vi "Add Default Enum.vi"(6 "Hdr Name":T1, 8 "error in (no error)":errorcluster, 9 "Enum Values":u16[](array[numeric]), 11 "Resistance in":refnum<class "Resistance.lvclass">) -> (0 "error out":errorcluster, 3 "Resistance out":refnum<class "Resistance.lvclass">)   [LabVIEW 2012, in "Measurement Channels.lvlib" / "Resistance.lvclass"]
uses:
  Resistance.lvclass
  Common/Controls/HeaderNames.ctl
  Resistance.lvclass/Resistance.ctl
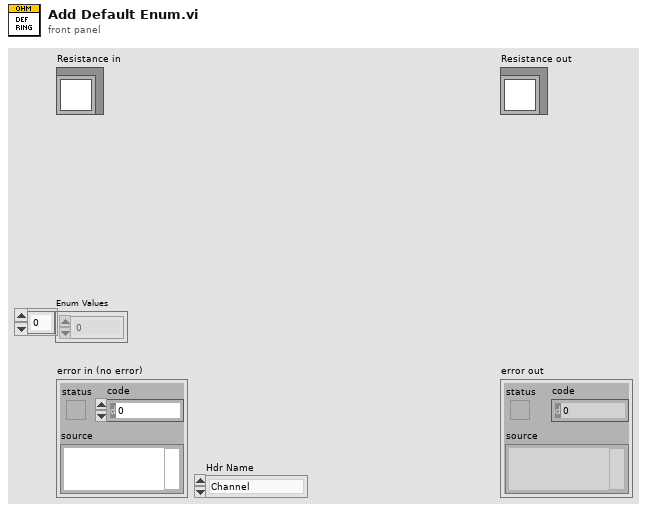
[diagram p1: front panel]
types:
  T1 = typedef "HeaderNames.ctl" = enum16{"Channel", "Device", "Spacer", "Description", "MB", "Range", "Terminal", "Coupling", "Thresh (V)", "Pulse/Rev", "Slope", "Min EU", "Min RPM", "mV/EU", "Iex", "Temp Units", "Type", "CJC Src", "CJC Val", "Ro", "Wire Cfg", "Strain Mode", "Vex", "Bridge Type", "GF", "Gauge Res", "Poisson", "Lead Res", "Init Strain", "GAF", "Scale", "Offset", "Unit (EU)", "dB?", "dB Ref", "Cal Mag", "Cal Units", "Max Temp", "Min Temp", "Max Strain", "Min Strain"}
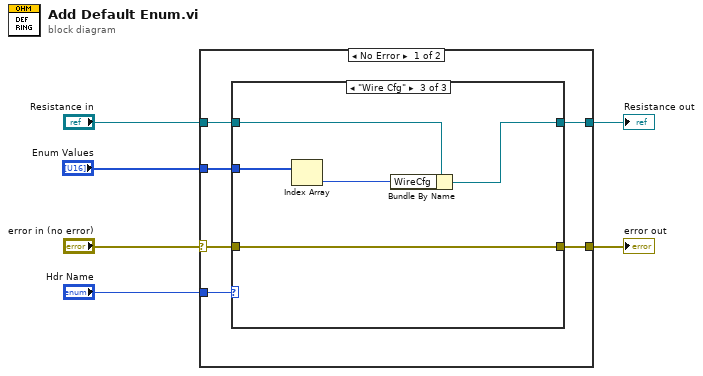
[diagram p0: block diagram]
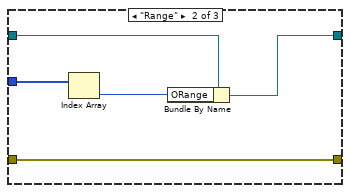
[diagram p3: hidden frame]
diagram:
  n1 = case shown="No Error" "error in (no error)" {
    selector: "error in (no error)" -> [w7 w26]
    tunnel: "Resistance in" -> [w12 w25]
    tunnel: "Enum Values" -> [w11 _]
    tunnel: [w10 w25] -> w2
    tunnel: "Hdr Name" -> [w9 _]
    tunnel: [w8 w26] -> w1
    frame No Error {
      n2 = case shown="\"Wire Cfg\"" w9 {
        tunnel: w12 -> [w14 w19 w24]
        tunnel: w11 -> [_ w18 w23]
        tunnel: [w14 w17 w22] -> w10
        tunnel: w7 -> [w13 w16 w21]
        tunnel: [w13 w16 w21] -> w8
        frame Default {
        }
        frame "Range" {
          n3 = Index Array(array=w18) -> (element=w15:u16)  [unwired: 1 in]
          n4 = Bundle By Name(cluster=w19, "ORange"=w15) -> (w17:refnum<class "Resistance.lvclass">)
        }
        frame "Wire Cfg" {
          n5 = Index Array(array=w23) -> (element=w20:u16)  [unwired: 1 in]
          n6 = Bundle By Name(cluster=w24, "WireCfg"=w20) -> (w22:refnum<class "Resistance.lvclass">)
        }
      }
    }
    frame Error {
    }
  }
  "error out" <- w1
  "Resistance out" <- w2
